vi "staticRFChannelUpdate.vi"(8 "error in (no error)":errorcluster, 10 "staticChannelUpdate":T1, 11 "AtomChipHWC in":refnum<class "AtomChipHWC.lvclass">) -> (0 "error out":errorcluster, 3 "AtomChipHWC out":refnum<class "AtomChipHWC.lvclass">)   [LabVIEW 2009, in "Hardware.lvlib" / "HWControllers.lvlib" / "AtomChipHWC.lvclass"]
uses:
  AtomChipHWC.lvclass
  AtomChipHWC.lvclass/AtomChipHWC.ctl
  Channels/DDSOutput/Generic/DDSOutput.lvclass
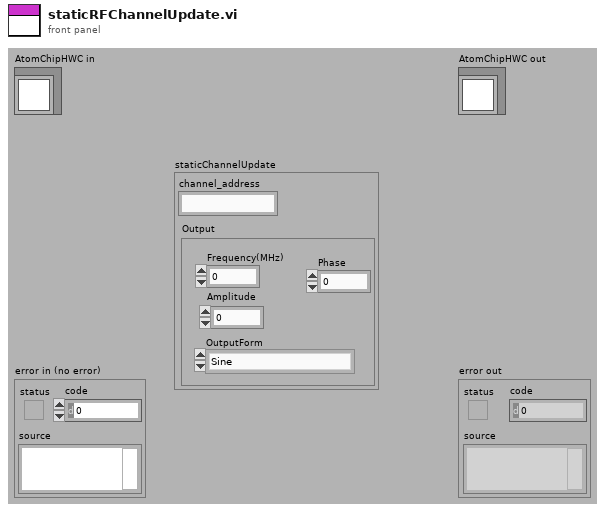
[diagram p1: front panel]
types:
  T1 = cluster{"channel_address":string, "Output":cluster{"Frequency(MHz)":dbl, "Amplitude":dbl, "Phase":dbl, "OutputForm":enum16{"Sine", "Square", "Triangle", "Arbitrary"}}}
  T2 = cluster{"Frequency(MHz)":dbl, "Amplitude":dbl, "Phase":dbl, "OutputForm":enum16{"Sine", "Square", "Triangle", "Arbitrary"}}
  T3 = cluster{"Frequency(MHz)":dbl, "Amplitude":dbl, "Phase":dbl, "OutputForm":enum16{"Sine", "Square", "Triangle", "Arbitrary"}}[]
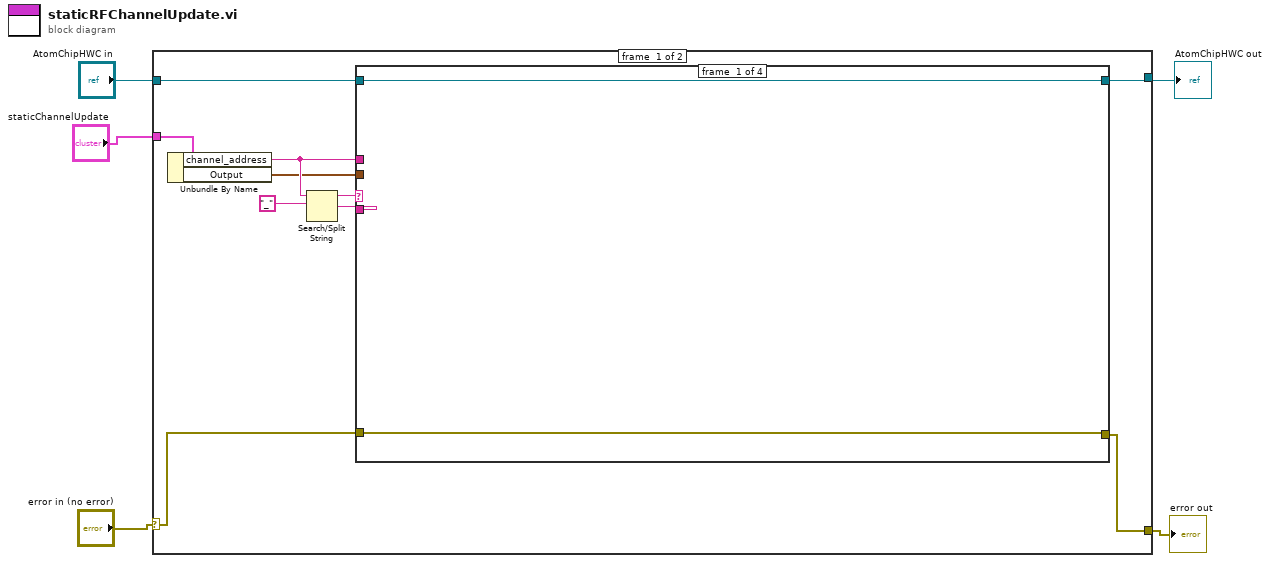
[diagram p0: block diagram]
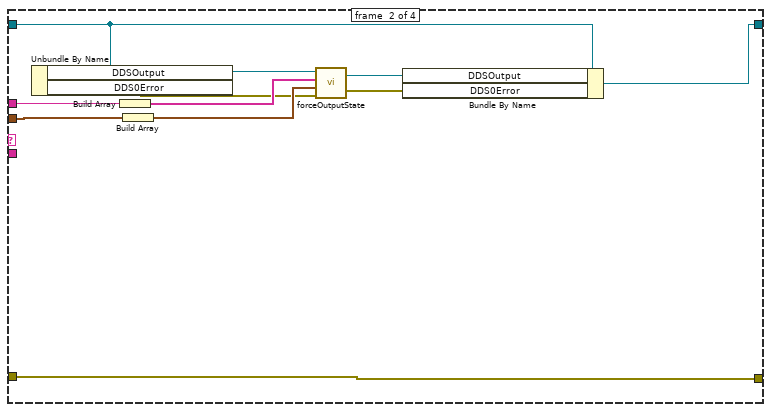
[diagram p2: hidden frame]
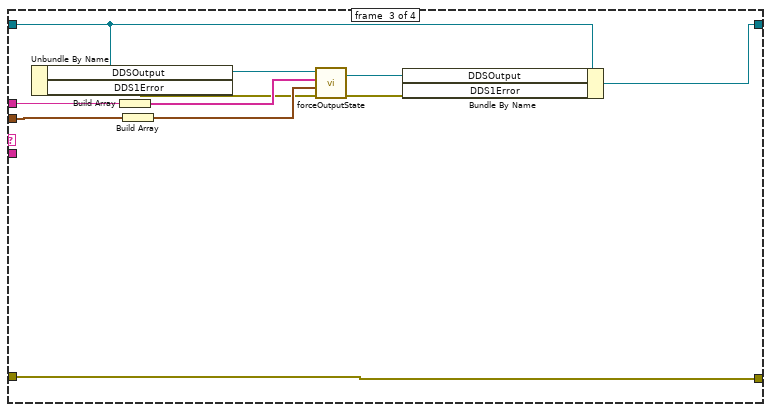
[diagram p3: hidden frame]
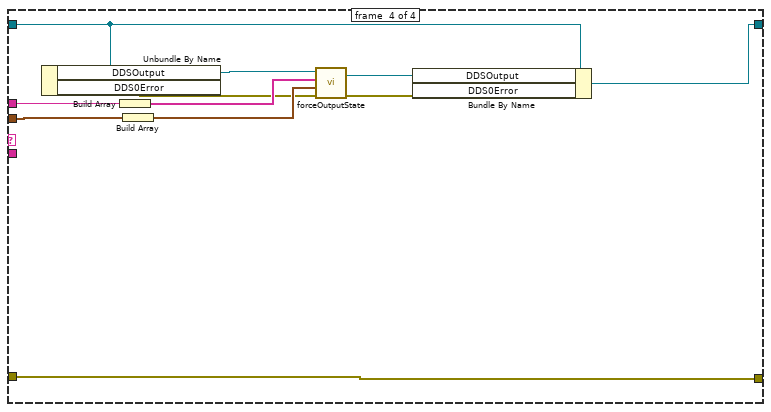
[diagram p4: hidden frame]
diagram:
  n1 = case shown="No Error" "error in (no error)" {
    selector: "error in (no error)" -> [w9 w51]
    tunnel: [w8 w51] -> w1
    tunnel: [w10 w52] -> w2
    tunnel: "AtomChipHWC in" -> [w11 w52]
    tunnel: "staticChannelUpdate" -> [w15 _]
    frame #0 {
      n2 = Unbundle By Name(w15) -> ("channel_address"=w12:string, "Output"=w7:T2)
      n3 = Search/Split String(string=w12, search string/char (-)="_") -> (substring before match=w13:string, match + rest of string=w6:string)  [unwired: 1 in, 1 out]
      n4 = case shown="\"CQTDDS0\"" w13 {
        tunnel: w12 -> [_ w27 w38 w49]
        tunnel: w11 -> [w17 w23 w34 w45]
        tunnel: [w17 w21 w32 w43] -> w10
        tunnel: w9 -> [w16 w18 w29 w40]
        tunnel: [w16 w18 w29 w40] -> w8
        tunnel: w7 -> [_ w25 w36 w47]
        tunnel: w6 -> [_ _ _ _]
        frame #0 {
        }
        frame #1 {
          n5 = Unbundle By Name(w23) -> ("DDSOutput"=w28:refnum<class "DDSOutput.lvclass">, "DDS0Error"=w20:errorcluster)
          n6 = Build Array(w27) -> (w26:string[])
          n7 = Build Array(w25) -> (w24:T3)
          n8 = call-dynamic "forceOutputState.vi"("error in (no error)"=w20, "data"=w24, "physicalChannels"=w26, "DDSOutput in"=w28) -> ("error out"=w19:errorcluster, "DDSOutput out"=w22:refnum<class "DDSOutput.lvclass">)  [unwired: 6 in]
          n9 = Bundle By Name(cluster=w23, "DDSOutput"=w22, "DDS0Error"=w19) -> (w21:refnum<class "AtomChipHWC.lvclass">)
        }
        frame #2 {
          n10 = Unbundle By Name(w34) -> ("DDSOutput"=w39:refnum<class "DDSOutput.lvclass">, "DDS1Error"=w31:errorcluster)
          n11 = Build Array(w38) -> (w37:string[])
          n12 = Build Array(w36) -> (w35:T3)
          n13 = call-dynamic "forceOutputState.vi"("error in (no error)"=w31, "data"=w35, "physicalChannels"=w37, "DDSOutput in"=w39) -> ("error out"=w30:errorcluster, "DDSOutput out"=w33:refnum<class "DDSOutput.lvclass">)  [unwired: 6 in]
          n14 = Bundle By Name(cluster=w34, "DDSOutput"=w33, "DDS1Error"=w30) -> (w32:refnum<class "AtomChipHWC.lvclass">)
        }
        frame #3 {
          n15 = Unbundle By Name(w45) -> ("DDSOutput"=w50:refnum<class "DDSOutput.lvclass">, "DDS0Error"=w42:errorcluster)
          n16 = Build Array(w49) -> (w48:string[])
          n17 = Build Array(w47) -> (w46:T3)
          n18 = call-dynamic "forceOutputState.vi"("error in (no error)"=w42, "data"=w46, "physicalChannels"=w48, "DDSOutput in"=w50) -> ("error out"=w41:errorcluster, "DDSOutput out"=w44:refnum<class "DDSOutput.lvclass">)  [unwired: 6 in]
          n19 = Bundle By Name(cluster=w45, "DDSOutput"=w44, "DDS0Error"=w41) -> (w43:refnum<class "AtomChipHWC.lvclass">)
        }
      }
    }
    frame #1 {
    }
  }
  "error out" <- w1
  "AtomChipHWC out" <- w2
